vi "Remote Control Receiver Loop.vi"() -> ()   [LabVIEW 2009]
uses:
  Remote Control/Control Message.ctl
  Remote Control/Motor Command.ctl
  Functional Global Variables/Actions for FG's.ctl
  UI Comm/Watchdog Dish Labels.ctl
panel:
  in  "Control Message":T1
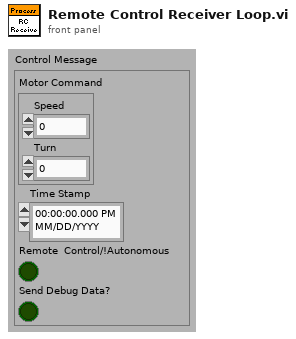
[diagram p1: front panel]
types:
  T1 = typedef "Control Message.ctl" = cluster{"Motor Command":T2, "Time Stamp":timestamp, "Remote  Control/!Autonomous":bool, "Send Debug Data?":bool}
  T2 = typedef "Motor Command.ctl" = cluster{"Speed":i16, "Turn":i16}
  T3 = typedef "UDP Base.ctl" = cluster{"UDP Session":refnum<k16>, "UDP Socket Params":T4}
  T4 = typedef "UDP Socket Params.ctl" = cluster{"Local Port":u16, "Read Timeout":i32, "Write Timeout":i32}
  T5 = typedef "Actions for FG's.ctl" = enum16{"Read", "Write"}
  T6 = typedef "Watchdog Dish Labels.ctl" = enum16{"GPS", "SICK", "Compass", "Cameras", "Motor Controller", "Debug", "RC Receiver"}
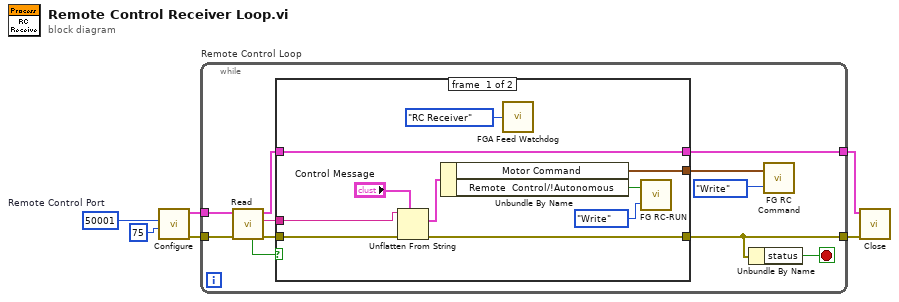
[diagram p0: block diagram]
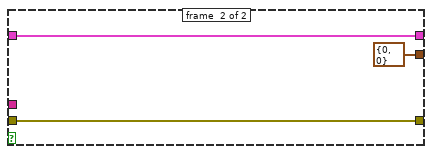
[diagram p2: hidden frame]
diagram:
  w2 = u16 50001  # Remote Control Port
  n1 = call "Configure.vi"("Read Timeout"=75, "Local Port"=w2) -> ("error out"=w5:errorcluster, "UDP Base out"=w6:T3)  [unwired: 8 in]
  n2 = while "Remote Control Loop" {
    tunnel: w6 -> [w15]
    tunnel: w5 -> [w14]
    tunnel: [w17] -> w3
    tunnel: [w16] -> w4
    stop <- w9 stop-if-true
    n3 = call "Read.vi"("error in (no error)"=w14, "UDP Base in"=w15) -> ("error out"=w12:errorcluster, "Receive Data"=w11:string, "UDP Base out"=w13:T3, "Timeout"=w10:bool)  [unwired: 4 in, 2 out]
    n4 = case shown="False" w10 {
      tunnel: [w21 w29] -> w17
      tunnel: [w22 w30] -> w16
      tunnel: w13 -> [w22 w30]
      tunnel: w12 -> [w26 w29]
      tunnel: w11 -> [w27 _]
      tunnel: [w19 T2 {"Speed"=0, "Turn"=0} ("Motor Command")] -> w8
      frame #0 {
        n5 = Unflatten From String(type="Control Message", binary string=w27, error in (no error)=w26) -> (value=w24:T1, error out=w21:errorcluster)  [unwired: 2 in, 1 out]
        n6 = Unbundle By Name(w24) -> ("Motor Command"=w19:T2, "Remote  Control/!Autonomous"=w23:bool)
        n7 = call "FGA Feed Watchdog.vi"("Watchdog Dish"=Watchdog_Dish_Labels."RC Receiver") -> ()  [unwired: 1 out]
        n8 = call "FG RC-RUN.vi"("FG Action (Read)"=Actions_for_FG's."Write" ("FG Action"), "RC/!Run in"=w23) -> ()  [unwired: 1 in, 1 out]
      }
      frame #1 {
      }
    }
    n9 = Unbundle By Name(w17) -> ("status"=w9:bool)
    n10 = call "FG RC Command.vi"("FG Action"=Actions_for_FG's."Write", "Motor Command in"=w8) -> ()  [unwired: 1 out]
  }
  n11 = call "Close.vi"("error in (no error)"=w3, "Cluster of class private data"=w4) -> ()  [unwired: 9 in, 1 out]
